vi "List tables.vi"(8 "error in (no error)":errorcluster, 11 "database":string) -> (0 "error out":errorcluster, 3 "tables":string[](array[string]))   [LabVIEW 2016, in "database.lvlib"]
uses:
  database.lvlib
  <vilib>/Utility/sysdir.llb/System Directory Type.ctl
  <vilib>/addons/database/Connection.llb/DB Tools Open Connec (String).vi
  <userlib>/_OpenG.lib/array/array.llb/Delete Elements from 1D Array (String)__ogtk.vi
  <vilib>/addons/database/NI_Database_API.lvlib
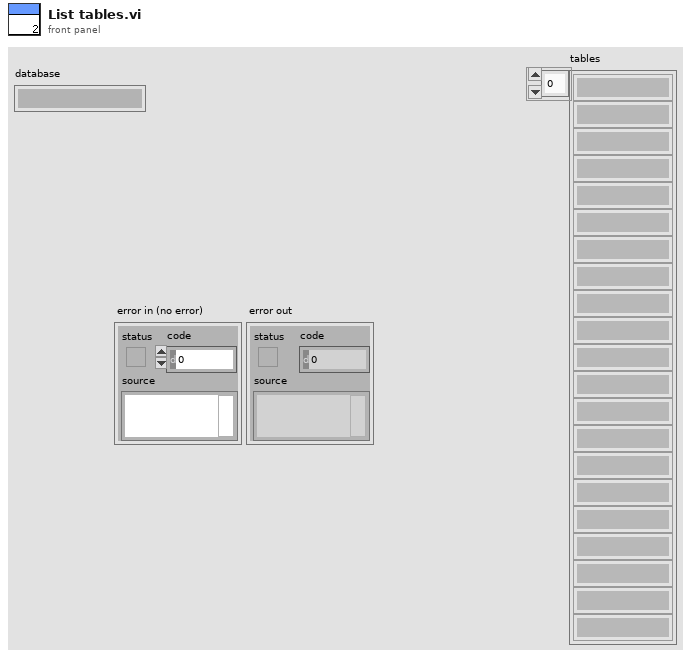
[diagram p1: front panel]
types:
  T1 = typedef "System Directory Type.ctl" = i32
  T2 = typedef "NI_Database_API.lvlib/Conn ObjectReference.ctl" = refnum<k1>
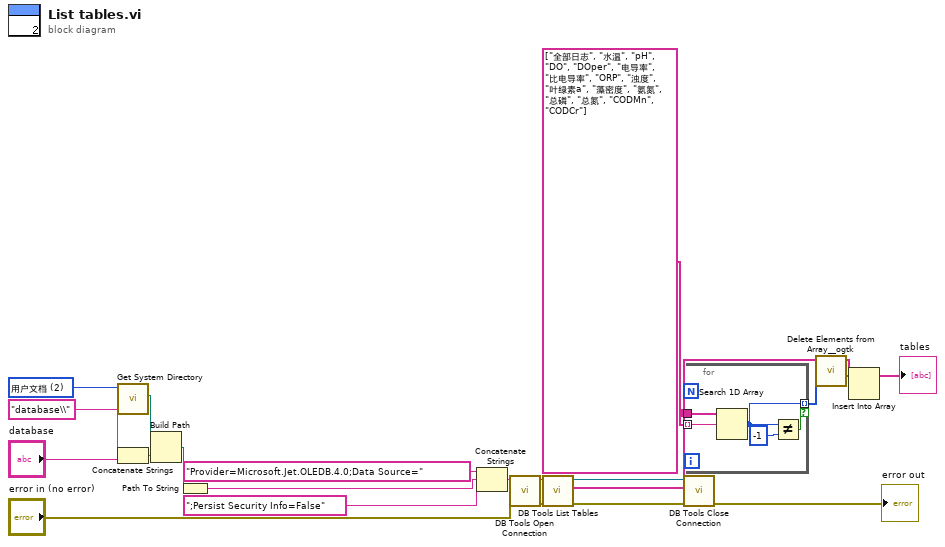
[diagram p0: block diagram]
diagram:
  w16 = T1 2 items=["用户目录"=0, "用户桌面"=1, "用户文档"=2, "用户应用程序数据"=3, "用户设置"=4, "用户临时目录"=5, "公共文档"=6, "公共应用程序数据"=7, "公共设置"=8, "公共缓存"=13, "系统核心库"=9, "系统安装库"=10, "应用程序文件"=11, "启动盘根目录"=12] ("system directory type")
  n1 = call <vilib>:"Get System Directory.vi"("system directory type"=w16) -> ("system directory"=w14:path)  [unwired: 10 in]
  n2 = Concatenate Strings("database\\" ("condition"), "database") -> (w8:string)
  n3 = Build Path(base path=w14, name or relative path=w8) -> (appended path=w13:path)
  n4 = Path To String(path=w13) -> (string=w12:string)
  n5 = Concatenate Strings("Provider=Microsoft.Jet.OLEDB.4.0;Data Source=" ("condition"), w12, ";Persist Security Info=False" ("condition")) -> (w10:string)
  n6 = call-poly <vilib>:"DB Tools Open Connection.vi"("error in (no error)"="error in (no error)", "connection information"=w10) -> ("error out"=w20:errorcluster, "connection reference"=w22:T2)  [unwired: 6 in]
  n7 = call <vilib>:"DB Tools List Tables.vi"("error in (no error)"=w20, "connection reference"=w22) -> ("error out"=w19:errorcluster, "tables"=w5:string[], "connection reference out"=w21:T2)  [unwired: 3 in]
  n8 = for {
    tunnel: w5 -> [w25]
    tunnel: string[] ["全部日志", "水温", "pH", "DO", "DOper", "电导率", "比电导率", "ORP", "浊度", "叶绿素a", "藻密度", "氨氮", "总磷", "总氮", "CODMn", "CODCr"] ("tables") -> [w27] mode=indexing
    tunnel: [w24] -> w4 mode=indexing if=w23
    n9 = Search 1D Array(1D array=w25, element=w27) -> (index of element=w24:i32)  [unwired: 1 in]
    n10 = Not Equal?(x=w24, y=-1) -> (x != y?=w23:bool)
  }
  n11 = call <vilib>:"DB Tools Close Connection.vi"("error in (no error)"=w19, "connection reference"=w21) -> ("error out"=→"error out":errorcluster)  [unwired: 5 in]
  n12 = call-poly <userlib>:"Delete Elements from Array__ogtk.vi"("indices"=w4, "array"=w5) -> ("deleted elements"=w3:string[], "array w/ subset deleted"=w2:string[])  [unwired: 8 in]
  n13 = Insert Into Array(array=w3, new element=w2) -> (→"tables":string[])  [unwired: 1 in]
